vi "Start Devices.vi"(8 "error in (no error)":errorcluster, 11 "Device Manager in":refnum<class "Device Manager.lvclass">) -> (0 "error out":errorcluster, 3 "Device Manager out":refnum<class "Device Manager.lvclass">)   [LabVIEW 2023, in "Device Manager.lvclass"]
uses:
  Device Manager.lvclass
  Device Manager.lvclass/Device Manager.ctl
  Device/Device Messages/Start Action Msg/Start Action Msg.lvclass
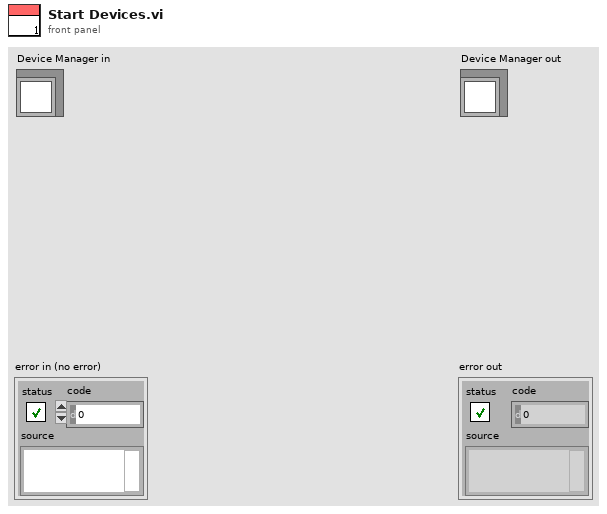
[diagram p1: front panel]
types:
  T1 = map{string, refnum<class "Message Enqueuer.lvclass">}
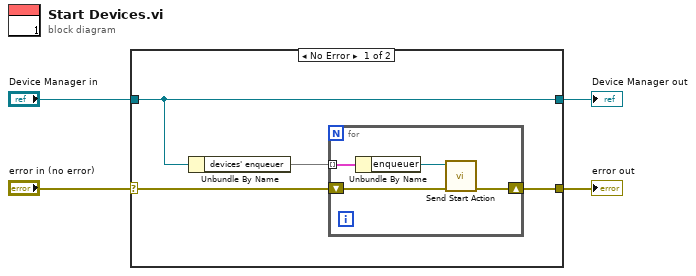
[diagram p0: block diagram]
diagram:
  n1 = case shown="No Error" "error in (no error)" {
    selector: "error in (no error)" -> [w8 w14]
    tunnel: [w6 w14] -> w3
    tunnel: [w7 w13] -> w1
    tunnel: "Device Manager in" -> [w7 w13]
    frame No Error {
      n2 = Unbundle By Name(w7) -> ("devices' enqueuer"=w5:T1)
      n3 = for {
        shift-right: [w11] -> w6
        shift-left: w8 -> [w12]
        tunnel: w5 -> [w10] mode=indexing
        n4 = Unbundle By Name(w10) -> ("enqueuer"=w9:refnum<class "Message Enqueuer.lvclass">)
        n5 = call "Send Start Action.vi"("error in (no error)"=w12, "Message Enqueuer"=w9) -> ("error out"=w11:errorcluster)  [unwired: 8 in, 1 out]
      }
    }
    frame Error {
    }
  }
  "error out" <- w3
  "Device Manager out" <- w1
